vi "Update Log.vi"(6 "Priority Message? (F)":bool, 8 "error in (no error)":errorcluster, 9 "Component":string="Archive", 10 "Status":string, 11 "UI Message Queue":refnum<queue>) -> (0 "error out":errorcluster, 2 "dup Status":string, 3 "dup UI Message Queue":refnum<queue>)   [LabVIEW 2024]
doc: "Adds a message to the back of a queue to update the running log."
uses:
  Shared/Message Queue/Message Cluster.ctl
  Controls/Server/Historical Log.ctl
  Shared/Message Queue.lvlib
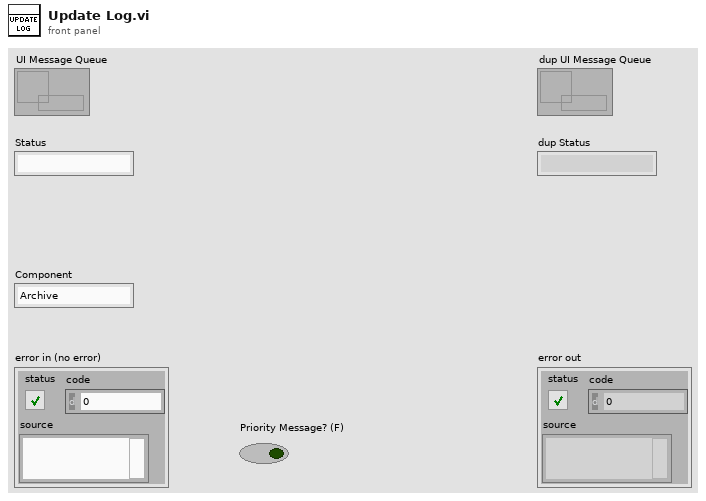
[diagram p1: front panel]
types:
  T1 = typedef "Historical Log.ctl" = cluster{"Time":timestamp, "Component":string, "Status":string}
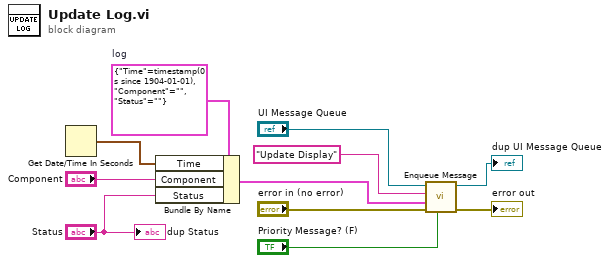
[diagram p0: block diagram]
diagram:
  w8 = T1 {"Time"=timestamp(0 s since 1904-01-01), "Component"="", "Status"=""}  # log
  n1 = Get Date/Time In Seconds() -> (seconds since 1Jan1904=w9:timestamp)
  n2 = Bundle By Name(cluster=w8, "Time"=w9, "Component"="Component", "Status"="Status") -> (w7:T1)
  n3 = call "Enqueue Message.vi"("Priority Message? (F)"="Priority Message? (F)", "error in (no error)"="error in (no error)", "Message Data"=w7, "Message"="Update Display", "Message Queue"="UI Message Queue") -> ("error out"=→"error out":errorcluster, "dup Message Queue"=→"dup UI Message Queue":refnum<queue>)  [unwired: 5 in]
  "dup Status" <- "Status"
